vi "Cam1Vision.vi"(0 "Image in":T1) -> (4 "方向正?针尖在右":bool, 5 "建坐标系OK":bool, 6 "Image Out":T1(plugin-control), 9 "数组":dbl[](array[numeric]))   [LabVIEW 2014]
uses:
  <vilib>/vision/Image Controls.llb/IMAQ Image.ctl
panel:
  out "Point1":cluster{"X":sgl, "Y":sgl}
  in  "选项卡控件":enum32{"选项卡 1", "选项卡 2", "选项卡 3"}(tab)
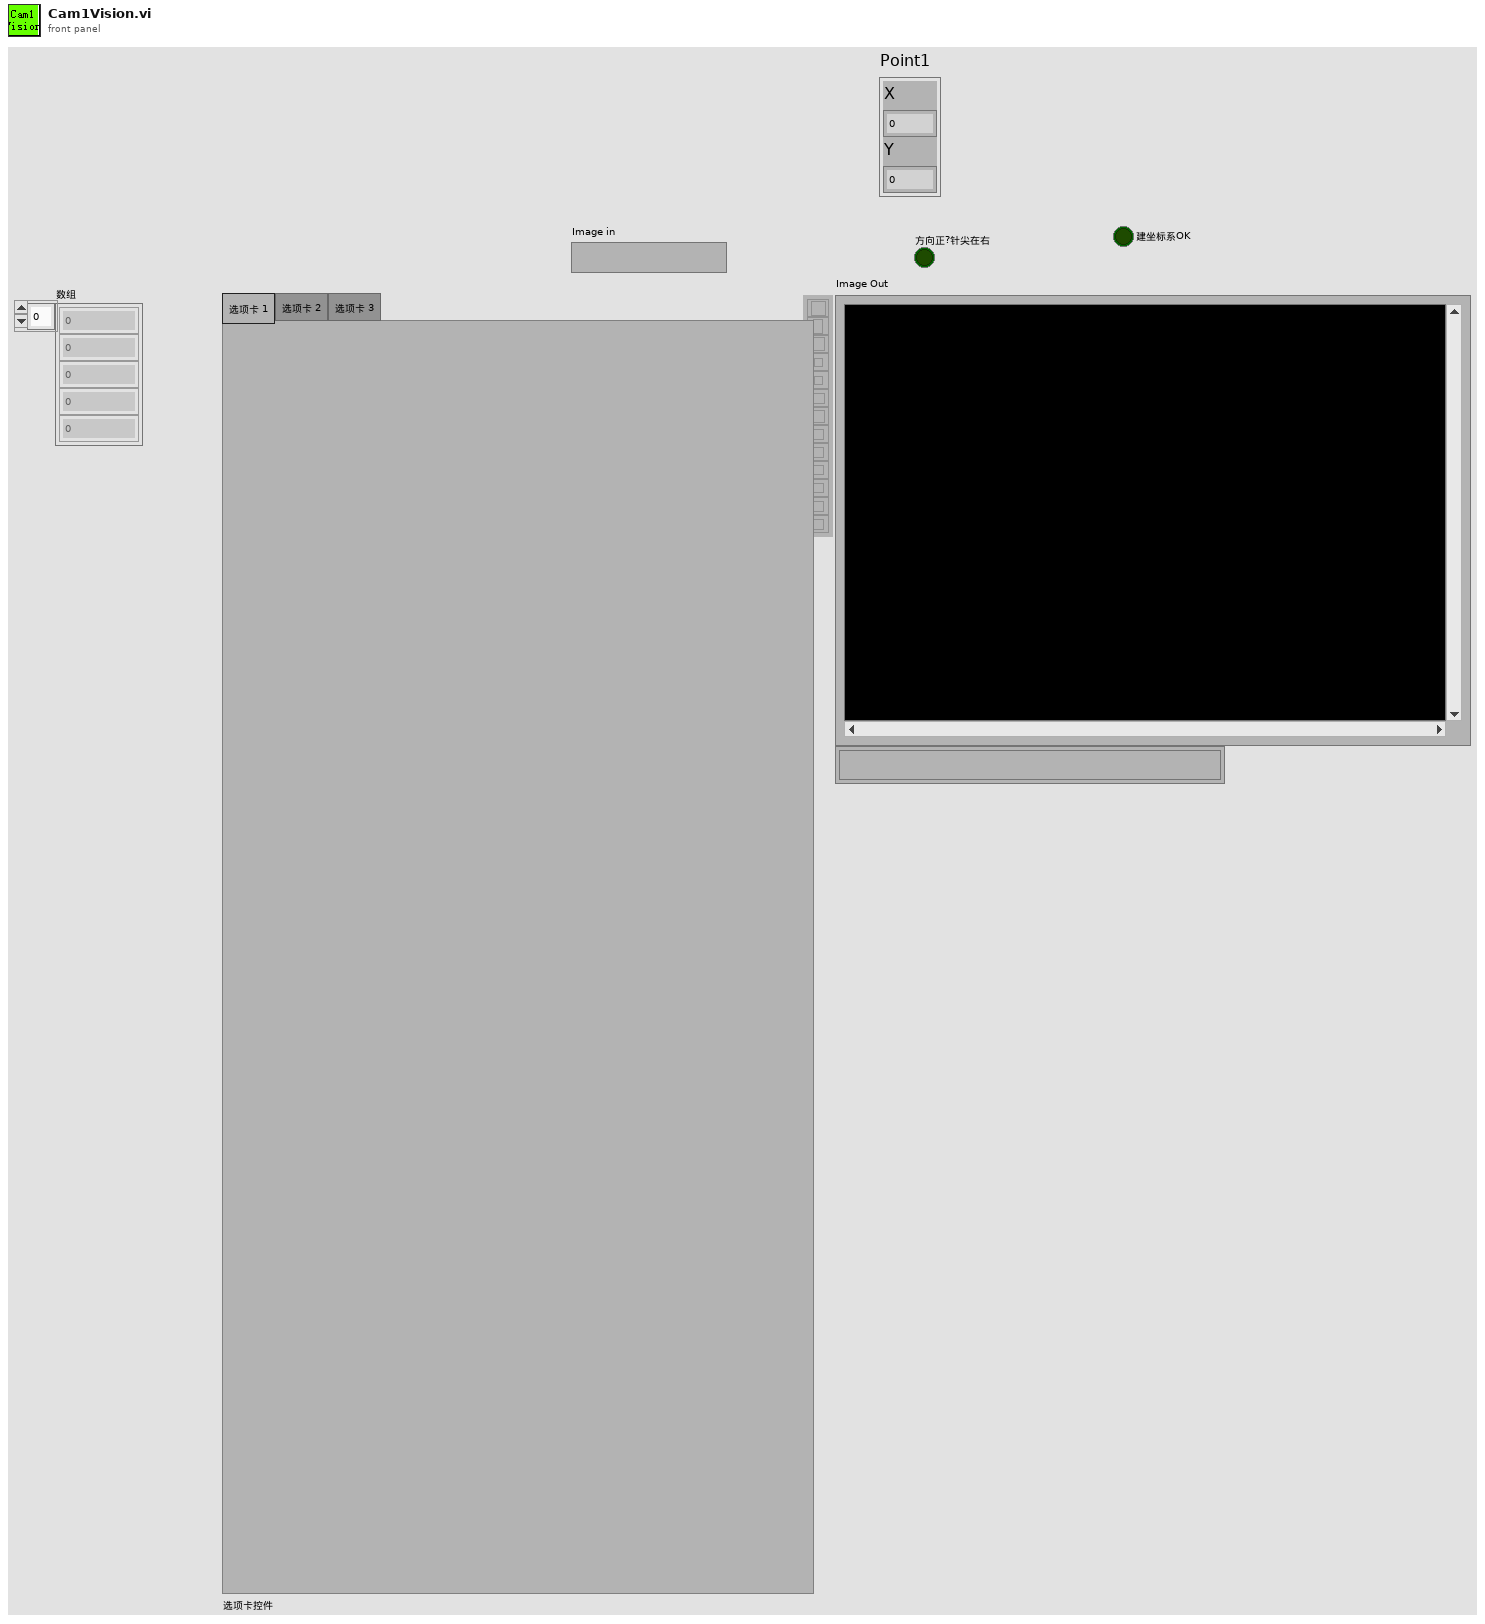
[diagram p1: front panel]
types:
  T1 = typedef "IMAQ Image.ctl" = refnum<image>
  T2 = cluster{"Point1 (Pixels)":cluster{"X":sgl, "Y":sgl}, "Point2 (Pixels)":cluster{"X":sgl, "Y":sgl}, "Point1 (Real-World)":cluster{"X":sgl, "Y":sgl}, "Point2 (Real-World)":cluster{"X":sgl, "Y":sgl}, "Angle (Pixel)":dbl, "Angle (Real-World)":dbl, "Score":dbl, "Straightness":dbl, "Average SNR (db)":dbl, "Calibration Valid":bool}
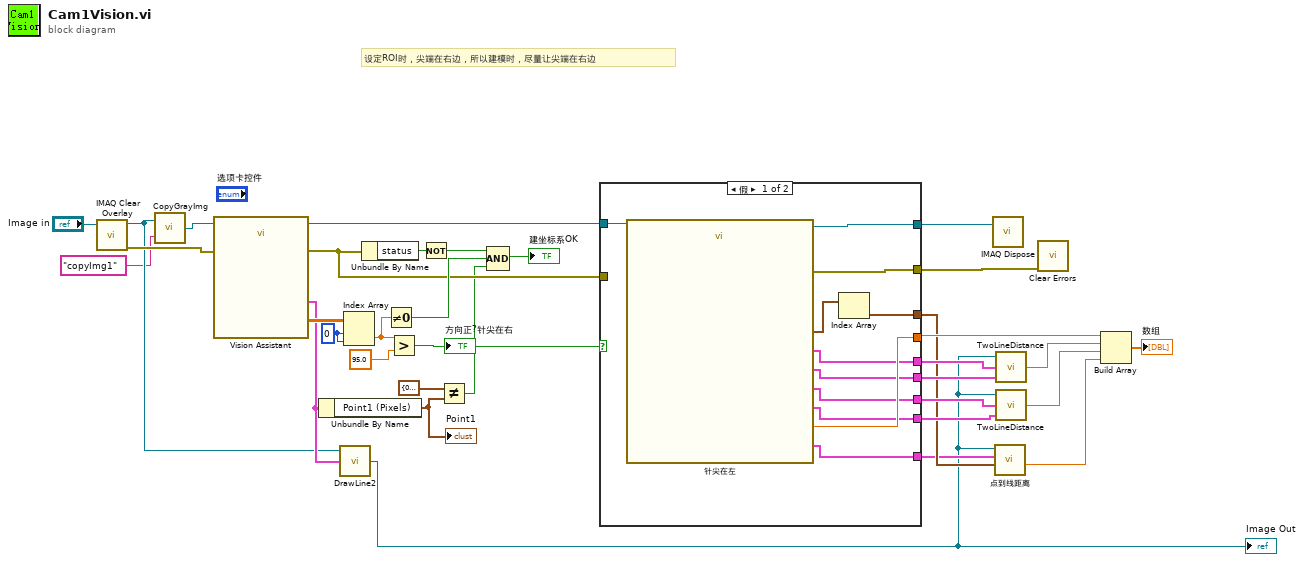
[diagram p0: block diagram]
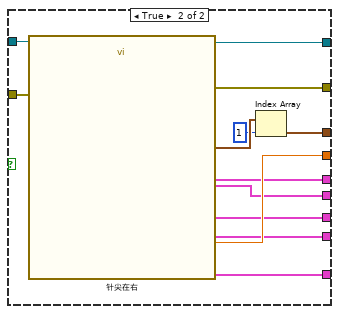
[diagram p2: hidden frame]
diagram:
  w30 = 0 ("索引 (行)")
  # "设定ROI时，尖端在右边，所以建模时，尽量让尖端在右边"
  n1 = call "IMAQ Clear Overlay"("Image"="Image in") -> ("error out"=w25:errorcluster, "Image Out"=w8:T1)  [unwired: 9 in]
  n2 = call "CopyGrayImg.vi"("Image Name"="copyImg1", "Image In"=w8) -> ("Image Out"=w6:T1)
  n3 = call "Vision Assistant"("Image In"=w6, "error in"=w25) -> ("Image Out"=w32:T1, "Caliper Results (Caliper 1)"=w31:sgl[][], "Straight Edge (FindX Edge)"=w9:T2, "error out"=w24:errorcluster)  [unwired: 22 in]
  n4 = Unbundle By Name(w9) -> ("Point1 (Pixels)"=w16:cluster{"X":sgl, "Y":sgl})
  "Point1" <- w16
  n5 = call "DrawLine2.vi"("输入簇"=w9, "img in"=w8) -> ("Image Out"=w2:T1)  [unwired: 1 in]
  "Image Out" <- w2
  n6 = Index Array(array=w31, index (row)=w30, index (col)=w30) -> (element=w27:sgl)
  n7 = Unbundle By Name(w24) -> ("status"=w29:bool)
  n8 = Not Equal To 0?(x=w27) -> (x != 0?=w26:bool)
  n9 = Greater?(x=w27, y=sgl 95.0) -> (0:w33:bool)
  "方向正?针尖在右" <- w33
  n10 = Not(x=w29) -> (.not. x?=w28:bool)
  n11 = Not Equal?(x=cluster{"X":sgl, "Y":sgl} {"X"=0.0, "Y"=0.0}, y=w16) -> (x != y?=w14:bool)
  n12 = Compound Arithmetic op=AND(w28, w26, w14) -> (→"建坐标系OK":bool)
  n13 = case shown="假" w33 {
    tunnel: w32 -> [w44 w57]
    tunnel: [w45 w58] -> w5
    tunnel: [w43 w56] -> w23
    tunnel: [w42 w55] -> w17
    tunnel: w24 -> [_ w54]
    tunnel: [w41 w53] -> w22
    tunnel: [w40 w52] -> w21
    tunnel: [w39 w51] -> w19
    tunnel: [w38 w50] -> w18
    tunnel: [w37 w49] -> w3
    tunnel: [w35 w47] -> w4
    frame False {
      n14 = call "针尖在左"("Image In"=w44, "Image Dst"=w44) -> ("Straight Edge (底部外径下直线)"=w38:T2, "Straight Edge (底部外径上直线)"=w39:T2, "Straight Edge (底部直线)"=w37:T2, "Image Out"=w45:T1, "Edge Coordinates (最左边点)"=w36:cluster{"X":sgl, "Y":sgl}[], "Distance (外环)"=w42:sgl, "Straight Edge (尖端外径上直线)"=w41:T2, "Straight Edge (尖端外径下直线)"=w40:T2, "error out"=w43:errorcluster)  [unwired: 17 in]
      n15 = Index Array(array=w36) -> (element=w35:cluster{"X":sgl, "Y":sgl})  [unwired: 1 in]
    }
    frame True {
      n16 = call "针尖在右"("Image In"=w57, "error in"=w54) -> ("Straight Edge (底部外径下直线)"=w50:T2, "Straight Edge (底部外径上直线)"=w51:T2, "Straight Edge (底部直线)"=w49:T2, "Image Out"=w58:T1, "Edge Coordinates (最左边点)"=w48:cluster{"X":sgl, "Y":sgl}[], "Distance (外环)"=w55:sgl, "Straight Edge (尖端外径上直线)"=w53:T2, "Straight Edge (尖端外径下直线)"=w52:T2, "error out"=w56:errorcluster)  [unwired: 17 in]
      n17 = Index Array(array=w48, index=1 ("索引")) -> (element=w47:cluster{"X":sgl, "Y":sgl})
    }
  }
  n18 = call "IMAQ Dispose"("Image"=w5) -> ()  [unwired: 5 in, 1 out]
  n19 = call "点到线距离.vi"("点坐标"=w4, "Straight Edge (Find Straight Edge 1)"=w3, "引用句柄输入"=w2) -> ("Distance"=w1:dbl)  [unwired: 7 in, 1 out]
  n20 = call "TwoLineDistance.vi"("外径下直线"=w21, "外径上直线"=w22, "Image in"=w2) -> ("Distance"=w20:dbl)
  n21 = call "TwoLineDistance.vi"("外径下直线"=w18, "外径上直线"=w19, "Image in"=w2) -> ("Distance"=w12:dbl)
  n22 = call <vilib>:"Clear Errors.vi"("error in (no error)"=w23) -> ()  [unwired: 5 in, 2 out]
  n23 = Build Array(w17, w20, w12, w1) -> (→"数组":dbl[])
